vi "_PC_D999 data_expand.vi"(1 "Refnum cluster in":T2) -> (0 "data cluster output":T1)   [LabVIEW 2018]
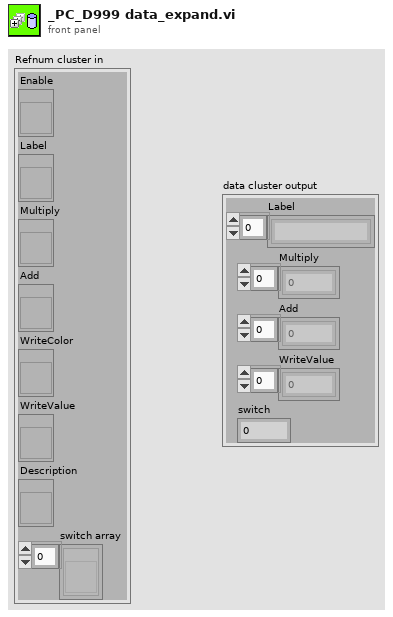
[diagram p1: front panel]
types:
  T1 = cluster{"Label":string[], "Multiply":dbl[], "Add":dbl[], "WriteValue":i16[], "switch":u32}
  T2 = cluster{"Enable":refnum<vi>, "Label":refnum<vi>, "Multiply":refnum<vi>, "Add":refnum<vi>, "WriteColor":refnum<vi>, "WriteValue":refnum<vi>, "Description":refnum<vi>, "switch array":refnum<vi>[]}
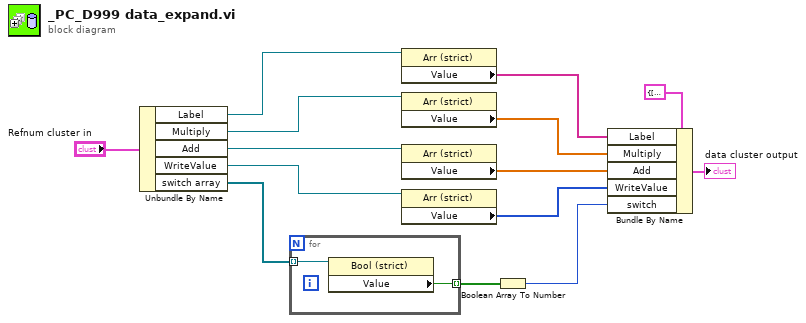
[diagram p0: block diagram]
diagram:
  n1 = Unbundle By Name("Refnum cluster in") -> ("Label"=w14:refnum<vi>, "Multiply"=w13:refnum<vi>, "Add"=w12:refnum<vi>, "WriteValue"=w11:refnum<vi>, "switch array"=w4:refnum<vi>[])
  n2 = for {
    tunnel: w4 -> [w16] mode=indexing
    tunnel: [w15] -> w3 mode=indexing
    n3 = property class="Bool (strict)"(reference=w16) -> ("Value"=w15:bool)  [unwired: 1 in, 2 out]
  }
  n4 = property class="Arr (strict)"(reference=w14) -> ("Value"=w6:string[])  [unwired: 1 in, 2 out]
  n5 = property class="Arr (strict)"(reference=w13) -> ("Value"=w7:dbl[])  [unwired: 1 in, 2 out]
  n6 = property class="Arr (strict)"(reference=w12) -> ("Value"=w8:dbl[])  [unwired: 1 in, 2 out]
  n7 = property class="Arr (strict)"(reference=w11) -> ("Value"=w9:i16[])  [unwired: 1 in, 2 out]
  n8 = Boolean Array To Number(Boolean array=w3) -> (number=w2:u32)
  n9 = Bundle By Name(cluster=T1 {"Label"=[], "Multiply"=[], "Add"=[], "WriteValue"=[], "switch"=0}, "Label"=w6, "Multiply"=w7, "Add"=w8, "WriteValue"=w9, "switch"=w2) -> (→"data cluster output":T1)
